vi "Clean Up.vi"(8 "error in (no error)":errorcluster, 11 "NIPKG Packager in":refnum<class "NIPKG Packager.lvclass">) -> (0 "error out":errorcluster)   [LabVIEW 2019, in "NIPKG Packager.lvclass"]
uses:
  NIPKG Packager.lvclass
  NIPKG Packager.lvclass/NIPKG Packager.ctl
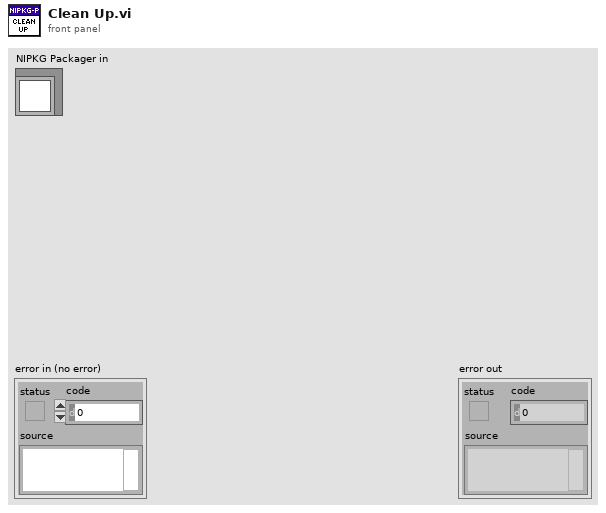
[diagram p1: front panel]
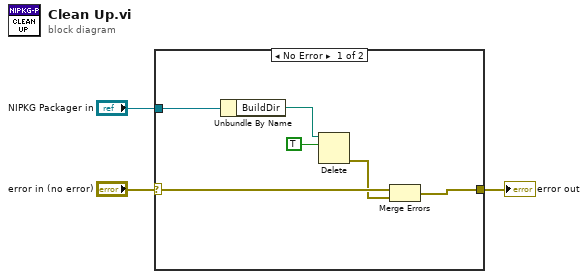
[diagram p0: block diagram]
diagram:
  n1 = case shown="No Error" "error in (no error)" {
    selector: "error in (no error)" -> [w9 w10]
    tunnel: [w5 w10] -> w2
    tunnel: "NIPKG Packager in" -> [w8 _]
    frame No Error {
      n2 = Unbundle By Name(w8) -> ("BuildDir"=w7:path)
      n3 = Delete(path (use dialog)=w7, entire hierarchy (F)=TRUE) -> (error out=w4:errorcluster)  [unwired: 3 in, 2 out]
      n4 = Merge Errors(w9, w4) -> (w5:errorcluster)
    }
    frame Error {
    }
  }
  "error out" <- w2
